vi "Pack for gRPC.vi"(8 "error in (no error)":errorcluster, 9 "Configuration / Resuls (Config)":enum16{"Configuration", "Results"}(ring), 10 "Data Value":variant, 11 "Measurement Customizations in":refnum<class "MeasurementPlugin.lvclass">) -> (0 "error out":errorcluster, 2 "Any":T1, 3 "Measurement Customizations out":refnum<class "MeasurementPlugin.lvclass">)   [LabVIEW 2021, in "Frequency Response_Audio ADC.lvlib" / "MeasurementPlugin.lvclass"]
uses:
  MeasurementPlugin.lvclass
  MeasurementPlugin.lvclass/MeasurementPlugin.ctl
  Measurement Configuration.ctl
  Frequency Response_Audio ADC.lvlib
  Measurement Results.ctl
  a6012965-5700-4384-8228-972e71b6560c.vi
  2eca732d-dbaa-43bf-a7dd-ede2da65bc1b.vi
  <vilib>/MeasurementLink/MeasurementLink Measurement Server/Measurement Plugin Service/Measurement Plugin Service.lvclass
  C:/Program Files/National Instruments/LabVIEW 2021/vi.lib/MeasurementLink/MeasurementLink Measurement Server/Measurement Plugin Service/Measurement Plugin Service.lvclass
  C:/community-repo/audio-adc-labview-add-plugin/source/frequency response/Frequency Response_Audio ADC/Advanced/MeasurementPlugin.lvclass
  <vilib>/gRPC/LabVIEW gRPC Library/Shared/Any.ctl
  <vilib>/gRPC/LabVIEW gRPC Library/grpc-lvsupport-release.lvlib
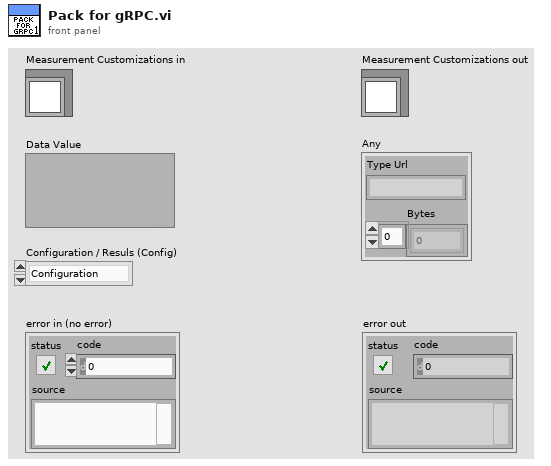
[diagram p1: front panel]
types:
  T1 = typedef "grpc-lvsupport-release.lvlib/Any.ctl" = cluster{"Type Url":string, "Bytes":u8[]}
  T2 = typedef "grpc-lvsupport-release.lvlib/grpcId.ctl" = u64
  T3 = typedef "Frequency Response_Audio ADC.lvlib/Measurement Configuration.ctl" = cluster{"Full scale range":dbl, "Maximum harmonic":i32, "Analog source resource name":string, "Frequency start":dbl, "Frequency stop":dbl, "Frequency steps":i32, "Frequency spacing":string, "Amplitude":dbl, "DC Offset":dbl, "Measurement duration":dbl, "Measurement cycles":i32, "Settling time":dbl, "Settling cycles":i32, "Protocol capture resource name":string, "Data line":u16, "Channel":u32, "Sample rate":dbl, "Frame sync edge for channel 0":u32, "Channel count per frame":u32, "Channel length":u32, "Bit depth":u32, "Channel 0 offset":u32, "Endianness":u32, "Data justification":u32, "Frame length":u32, "Frame sync pulse width":u32, "Bit clock edge sync":u32}
  T4 = typedef "Frequency Response_Audio ADC.lvlib/Measurement Results.ctl" = cluster{"Frequency steps":dbl[], "Frequency response":dbl[], "RMS levels":dbl[], "THD response":dbl[], "THD+N response":dbl[], "dt":dbl, "Time domain plot sizes":i32[], "Time domain":dbl[]}
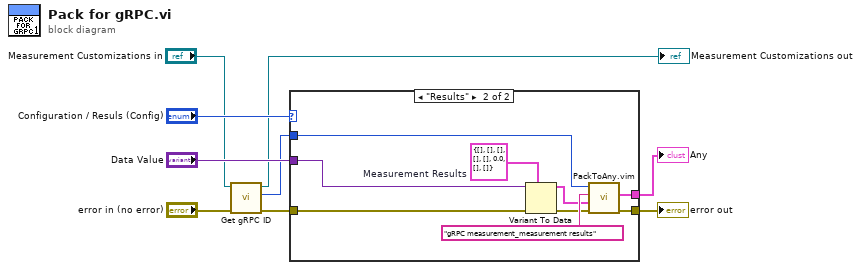
[diagram p0: block diagram]
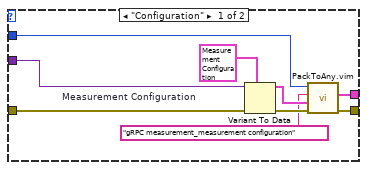
[diagram p2: hidden frame]
diagram:
  n1 = call <vilib>:"Get gRPC ID.vi"("error in"="error in (no error)", "measurement plugin service in"="Measurement Customizations in") -> ("error out"=w4:errorcluster, "gRPC ID"=w1:T2, "measurement plugin service out"=→"Measurement Customizations out":refnum<class "MeasurementPlugin.lvclass">)  [unwired: 7 in]
  n2 = case shown="\"Results\"" "Configuration / Resuls (Config)" {
    tunnel: w4 -> [w18 w27]
    tunnel: "Data Value" -> [w17 w26]
    tunnel: w1 -> [w14 w22]
    tunnel: [w16 w24] -> w8
    tunnel: [w15 w23] -> w7
    frame "Configuration" {
      w11 = T3 {"Full scale range"=3.16, "Maximum harmonic"=5, "Analog source resource name"="", "Frequency start"=100.0, "Frequency stop"=20000.0, "Frequency steps"=50, "Frequency spacing"="", "Amplitude"=1.0, "DC Offset"=0.0, "Measurement duration"=0.001, "Measurement cycles"=10, "Settling time"=0.0, "Settling cycles"=0, "Protocol capture resource name"="", "Data line"=0, "Channel"=0, "Sample rate"=12288000.0, "Frame sync edge for channel 0"=1, "Channel count per frame"=2, "Channel length"=32, "Bit depth"=24, "Channel 0 offset"=1, "Endianness"=0, "Data justification"=0, "Frame length"=64, "Frame sync pulse width"=32, "Bit clock edge sync"=1}  # Measurement Configuration
      n3 = Variant To Data(error in=w18, type=w11, Variant=w17) -> (data=w13:T3, error out=w12:errorcluster)
      n4 = call "PackToAny.vim"("error in"=w12, "Data To Pack"=w13, "Message Type"="gRPC measurement_measurement configuration", "gRPCid in"=w14) -> ("error out"=w16:errorcluster, "Any"=w15:T1)  [unwired: 5 in, 1 out]
    }
    frame "Results" {
      w25 = T4 {"Frequency steps"=[], "Frequency response"=[], "RMS levels"=[], "THD response"=[], "THD+N response"=[], "dt"=0.0, "Time domain plot sizes"=[], "Time domain"=[]}  # Measurement Results
      n5 = Variant To Data(error in=w27, type=w25, Variant=w26) -> (data=w20:T4, error out=w19:errorcluster)
      n6 = call "PackToAny.vim"("error in"=w19, "Data To Pack"=w20, "Message Type"="gRPC measurement_measurement results", "gRPCid in"=w22) -> ("error out"=w24:errorcluster, "Any"=w23:T1)  [unwired: 5 in, 1 out]
    }
  }
  "error out" <- w8
  "Any" <- w7
